vi "Timer data class VI - timer mechanics.vi"(8 "error in (no error)":errorcluster, 11 "Timer in":refnum<class "Timer.lvclass">) -> (0 "error out":errorcluster, 2 "elapsed time (milliseconds)":u32, 3 "Timer out":refnum<class "Timer.lvclass">)   [LabVIEW 2010, in "Timer.lvclass"]
uses:
  Timer.lvclass
panel:
  out "Enum":enum16{"Idle", "Start", "Continue", "Reset"}(ring)
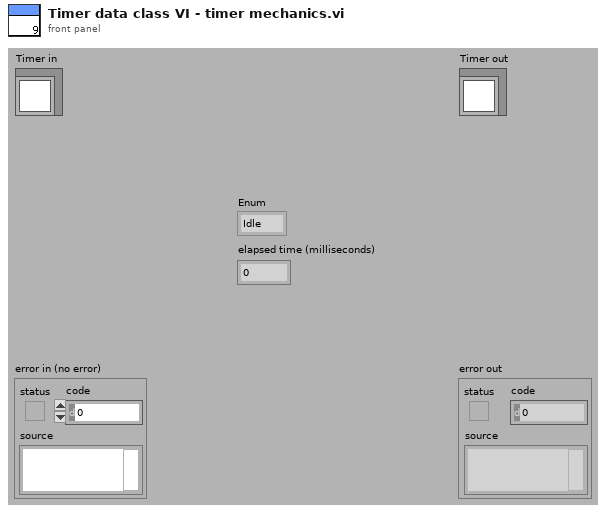
[diagram p1: front panel]
types:
  T1 = typedef "Timing Control.ctl" = enum16{"Idle", "Start", "Continue", "Reset"}
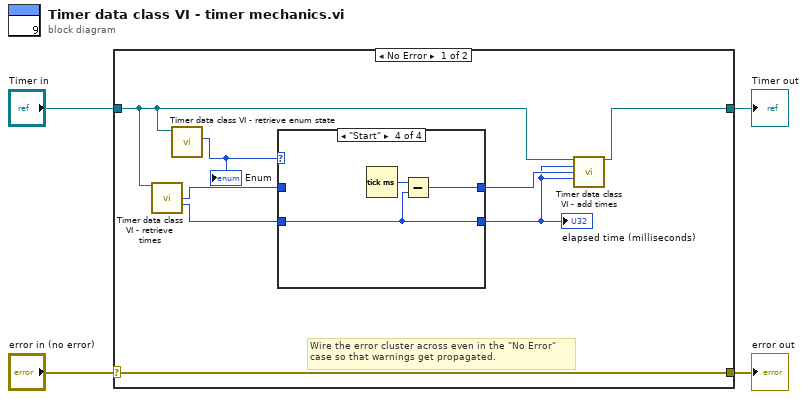
[diagram p0: block diagram]
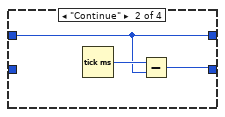
[diagram p3: hidden frame]
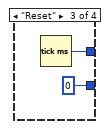
[diagram p4: hidden frame]
diagram:
  n1 = case shown="No Error" "error in (no error)" {
    selector: "error in (no error)" -> [w12 w24]
    tunnel: [w12 w24] -> w3
    tunnel: [w11 w23] -> w1
    tunnel: "Timer in" -> [w6 w23]
    frame No Error {
      # "Wire the error cluster across even in the \"No Error\"\ncase so that warnings get propagated."
      n2 = call-dynamic "Timer data class VI - retrieve times.vi"("Timer in"=w6) -> ("Time 1"=w9:u32, "Time 2"=w10:u32)  [unwired: 10 in, 3 out]
      n3 = call-dynamic "Timer data class VI - retrieve enum state.vi"("Timer in"=w6) -> ("State"=w5:T1)  [unwired: 8 in, 2 out]
      "Enum" <- w5
      n4 = case shown="\"Start\"" w5 {
        tunnel: [w13 w15 u32 0 w20] -> w7
        tunnel: [w14 w16 w18 w22] -> w8
        tunnel: w9 -> [w14 w16 _ _]
        tunnel: w10 -> [w13 _ _ w20]
        frame "Idle", Default {
        }
        frame "Continue" {
          n5 = Tick Count (ms)() -> (millisecond timer value=w17:u32)
          n6 = Subtract(x=w17, y=w16) -> (x-y=w15:u32)
        }
        frame "Reset" {
          n7 = Tick Count (ms)() -> (millisecond timer value=w18:u32)
        }
        frame "Start" {
          n8 = Tick Count (ms)() -> (millisecond timer value=w21:u32)
          n9 = Subtract(x=w21, y=w20) -> (x-y=w22:u32)
        }
      }
      "elapsed time (milliseconds)" <- w7
      n10 = call-dynamic "Timer data class VI - add times.vi"("Timer in"=w6, "Milliseconds"=w7, "Time 1"=w8, "Time 2"=w7) -> ("Timer out"=w11:refnum<class "Timer.lvclass">)  [unwired: 10 in, 1 out]
    }
    frame Error {
    }
  }
  "error out" <- w3
  "Timer out" <- w1
